vi "File Scan Values.vi"(10 "parameter vals scanned":dbl[](array[numeric]), 11 "values to scan":dbl[](array[numeric])) -> (1 "Quit":bool, 2 "shotgraph":cluster{"Output Array":dbl[], i32[]}, 3 "next value":dbl)   [LabVIEW 2013]
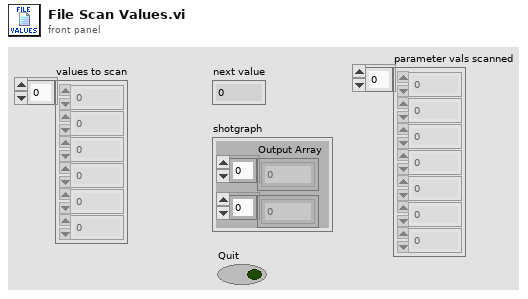
[diagram p1: front panel]
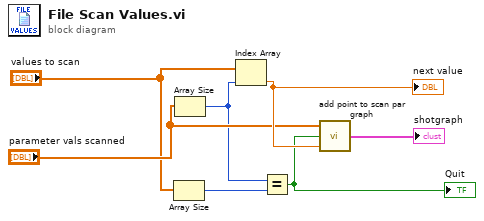
[diagram p0: block diagram]
diagram:
  n1 = Array Size(array="values to scan") -> (size(s)=w4:i32)
  n2 = Array Size(array="parameter vals scanned") -> (size(s)=w3:i32)
  n3 = Index Array(array="values to scan", index=w3) -> (element=w6:dbl)
  "next value" <- w6
  n4 = Equal?(x=w3, y=w4) -> (x = y?=w1:bool)
  "Quit" <- w1
  n5 = call "add point to scan par graph.vi"("next scan val"=w6, "scan complete"=w1, "shot times"="parameter vals scanned") -> ("shotgraph"=→"shotgraph":cluster{"Output Array":dbl[], i32[]})
